vi "2024_day10.vi"() -> ()   [LabVIEW 2023]
uses:
  <userlib>/_OpenG.lib/string/string.llb/openg_string.lvlib
  <userlib>/_OpenG.lib/array/array.llb/openg_array.lvlib
  <userlib>/_OpenG.lib/array/array.llb/Search 1D Array (I32)__ogtk.vi
panel:
  out "number":i32[][](array[numeric])
  in  "Switch":bool caption="Ex. Data  vs.  User Data"
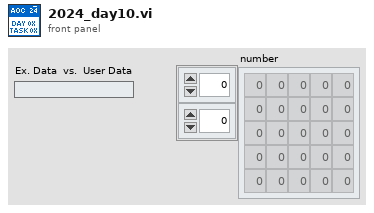
[diagram p1: front panel]
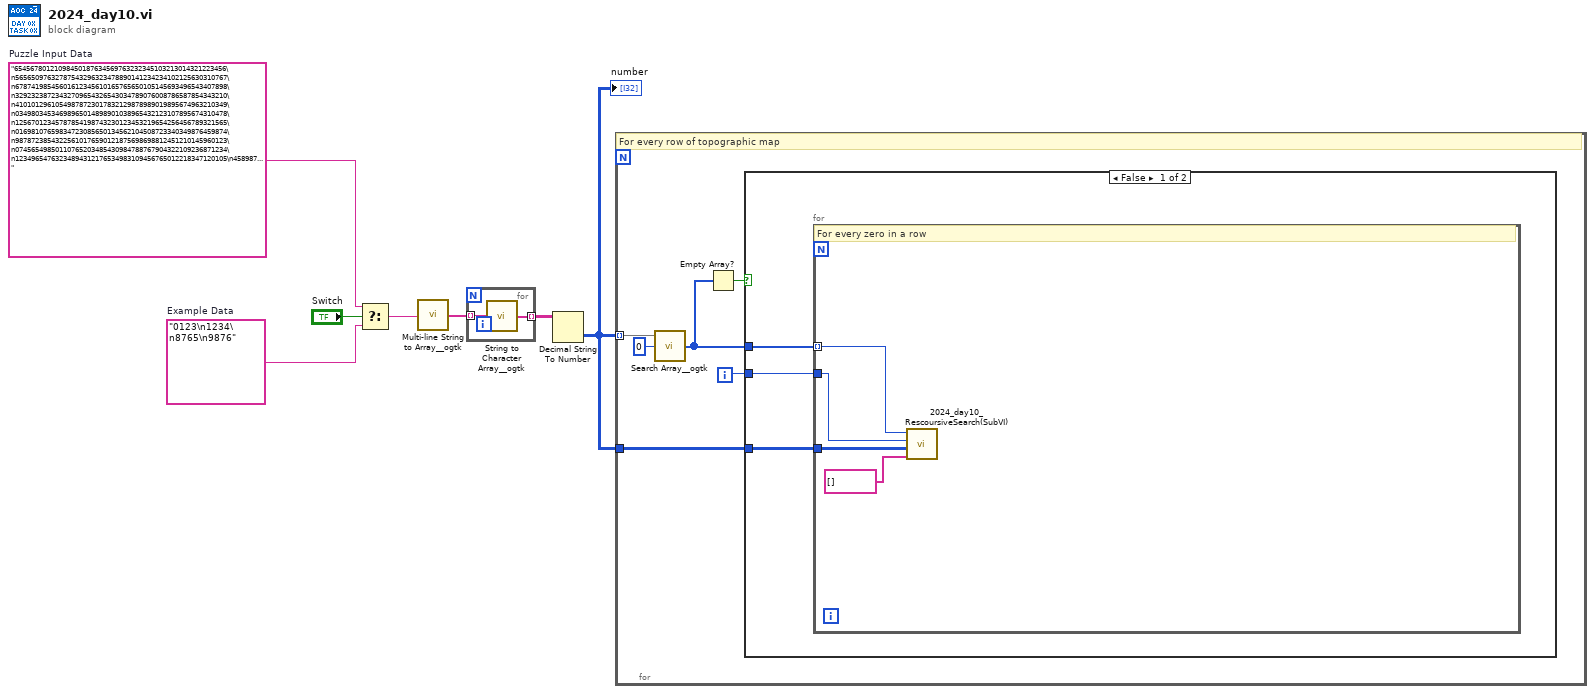
[diagram p0: block diagram]
diagram:
  w5 = "65456780121098450187634569763232345103213014321223456\n56565097632787543296323478890141234234102125630310767\n67874198545601612345610165765650105145693496543407898\n32923238723432709654326543034789076008786587854343210\n41010129610549878723017832129878989019895674963210349\n03498034534698965014898901038965432123107895674310478\n12567012345787854198743230123453219654256456789321565\n01698107659834723085650134562104508723340349876459874\n98787238543225610176590121875698698812451210145960123\n07456549850110765203485430984788767904322109236871234\n12349654763234894312176534983109456765012218347120105\n458987..."  # Puzzle Input Data
  w6 = "0123\n1234\n8765\n9876"  # Example Data
  n1 = Select(t=w5, s="Switch", f=w6) -> (s? t:f=w4:string)
  n2 = call <userlib>:"Multi-line String to Array__ogtk.vi"("string"=w4) -> ("lines"=w3:string[])
  n3 = for {
    tunnel: w3 -> [w9] mode=indexing
    tunnel: [w8] -> w2 mode=indexing
    n4 = call <userlib>:"String to Character Array__ogtk.vi"("Input String"=w9) -> ("Character Array"=w8:string[])
  }
  n5 = Decimal String To Number(string=w2) -> (number=w1:i32[][])  [unwired: 2 in, 1 out]
  "number" <- w1
  n6 = for {
    tunnel: w1 -> [w15] mode=indexing
    tunnel: w1 -> [w10]
    i -> [w11]
    # "For every row of topographic map"
    n7 = call-poly <userlib>:"Search Array__ogtk.vi"("Array"=w15, "Element Data"=0) -> ("Indices of Elements"=w12:i32[])  [unwired: 7 in]
    n8 = Empty Array?(array=w12) -> (empty?=w13:bool)
    n9 = case shown="False" w13 {
      tunnel: w12 -> [w18 _]
      tunnel: w11 -> [w17 _]
      tunnel: w10 -> [w16 _]
      frame False {
        n10 = for {
          tunnel: w18 -> [w21] mode=indexing
          tunnel: w17 -> [w22]
          tunnel: w16 -> [w20]
          # "For every zero in a row"
          n11 = call "2024_day10_RescoursiveSearch(SubVI).vi"("Trailheads In"=string[] [], "Topographic Map"=w20, "Start Column"=w22, "Start Row"=w21) -> ()  [unwired: 7 in, 1 out]
        }
      }
      frame True {
        # "No zeros in this line"
      }
    }
  }
